vi "Write LS DAQ Task.vi"(8 "error in (no error)":errorcluster, 10 "Data Acquisition.lvlib:DAQ Task.lvclass":refnum<class "DAQ Task.lvclass">, 11 "Chassis Tasks in":refnum<class "Chassis Tasks.lvclass">) -> (0 "error out":errorcluster, 3 "Chassis Tasks out":refnum<class "Chassis Tasks.lvclass">)   [LabVIEW 2018, in "Data Acquisition.lvlib" / "Chassis Tasks.lvclass"]
uses:
  Chassis Tasks.lvclass
  Class DAQ Task/DAQ Task.lvclass
  Chassis Tasks.lvclass/Chassis Tasks.ctl
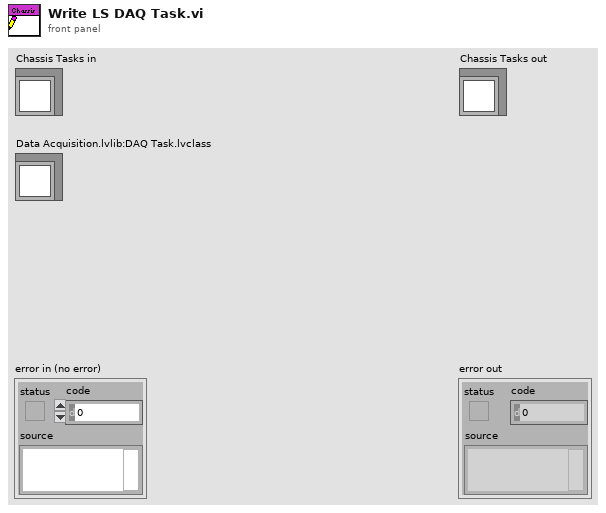
[diagram p1: front panel]
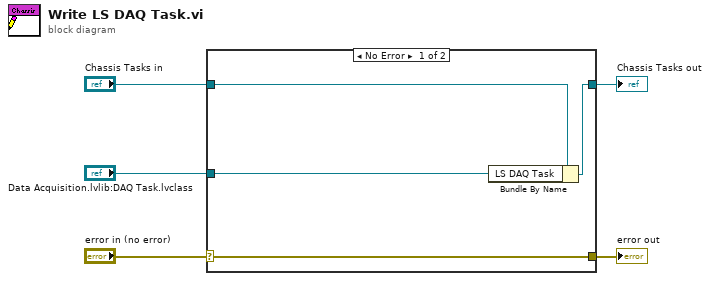
[diagram p0: block diagram]
diagram:
  n1 = case shown="No Error" "error in (no error)" {
    selector: "error in (no error)" -> [w9 w10]
    tunnel: [w9 w10] -> w4
    tunnel: [w7 w11] -> w2
    tunnel: "Chassis Tasks in" -> [w8 w11]
    tunnel: "Data Acquisition.lvlib:DAQ Task.lvclass" -> [w6 _]
    frame No Error {
      n2 = Bundle By Name(cluster=w8, "LS DAQ Task"=w6) -> (w7:refnum<class "Chassis Tasks.lvclass">)
    }
    frame Error {
    }
  }
  "error out" <- w4
  "Chassis Tasks out" <- w2
